vi "Analog Current Input - 1 Channel - Continuous Sampling.vi"() -> ()   [LabVIEW 2019]
uses:
  <vilib>/myRIO/Common/Instrument Driver Framework/myRIO v1.0/UART/vis/myRIO v1.0 Close UART.vi
  <vilib>/myRIO/Instrument Drivers/Onboard IO/AI Continuous/vis/AI Continuous Smart Read.vi
  <vilib>/myRIO/Common/Instrument Driver Framework/Utilities/vis/FPGA Ref Manager.vi
  <vilib>/myRIO/Common/Instrument Driver Framework/ELVIS III v1.0/ELVIS III v1.0 Reset FPGA.vi
  <vilib>/myRIO/Common/Instrument Driver Framework/myRIO v1.0/IRQ/vis/myRIO v1.0 IRQ Info FGV.vi
  <vilib>/myRIO/Common/Instrument Driver Framework/myRIO v1.0/IRQ/vis/myRIO v1.0 Timer IRQ Info FGV.vi
  <vilib>/myRIO/Common/Instrument Driver Framework/myRIO v1.0/IRQ/vis/myRIO v1.0 ISR Agent.vi
  <vilib>/myRIO/Instrument Drivers/Utilities/vis/Reset Index.vi
  <vilib>/myRIO/Common/Instrument Driver Framework/myRIO v1.0/Resource Manager/vis/myRIO v1.0 Block Write Resource Manager.vi
  <vilib>/myRIO/Express VI/Onboard IO/AI/AI Express VI.xnode
  <vilib>/myRIO/Instrument Drivers/Utilities/Utilities.lvlib
  <vilib>/myRIO/Instrument Drivers/Onboard IO/AI Continuous/AI Continuous.lvlib
panel:
  in  "电阻数值":dbl=1000.0 format="%#_6p"
  out "Analog Data":dbl[](graph)
  in  "Stop":bool
  # "ELVIS III Control IO"
  # "模拟输入单通道连续采样"
  # "Overview: Acquires current values continuously from Bank A, Channel 0 (A/AI0) until the acquisition is stopped.\nInstructions:\n1. Connect A/AI0 to a valid signal.\n2. Run the VI."
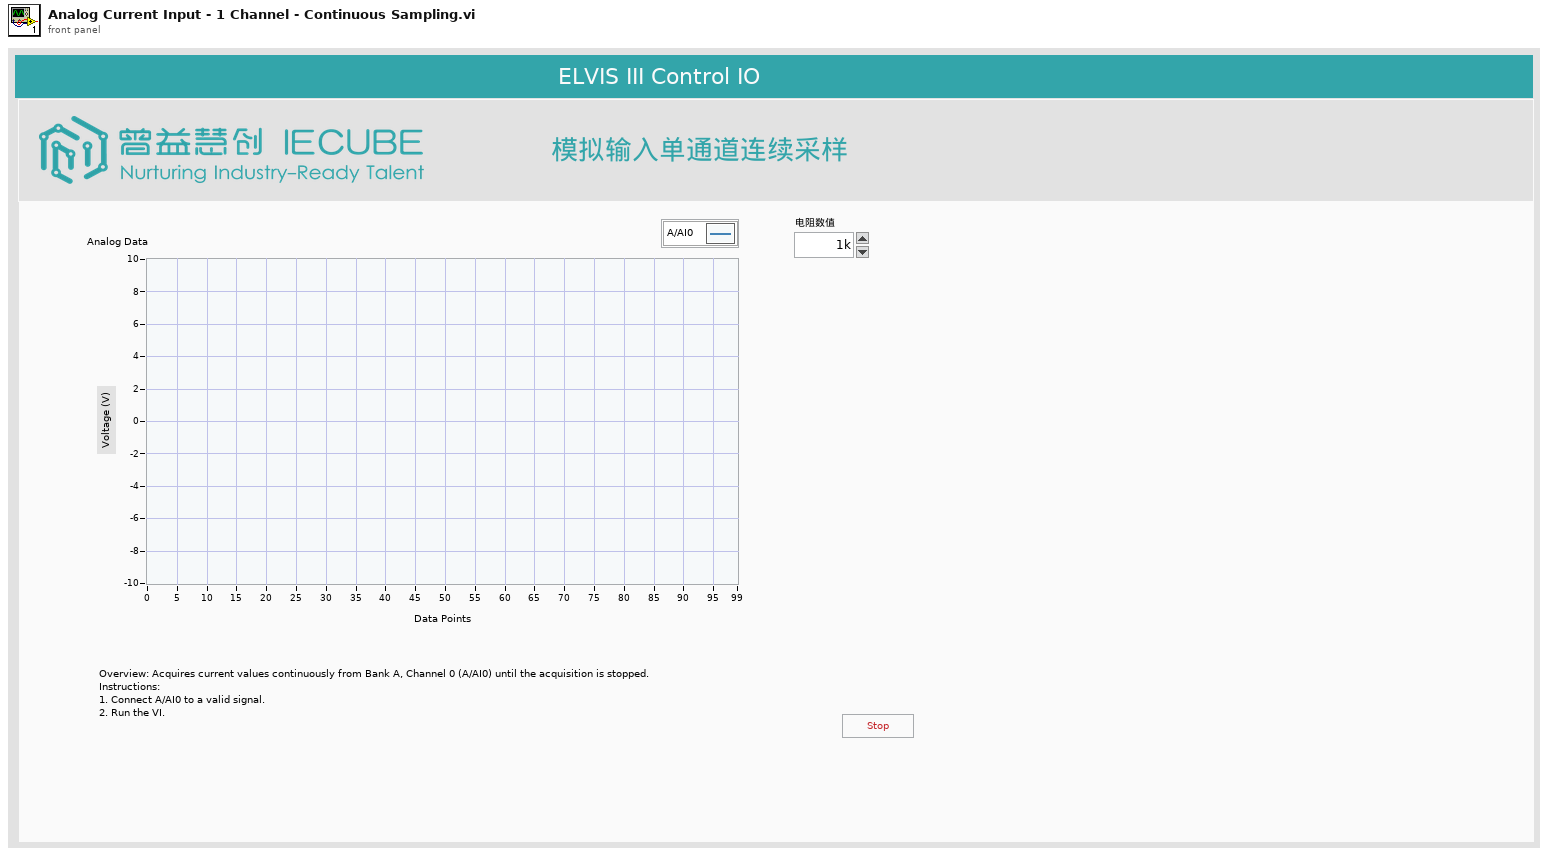
[diagram p1: front panel]
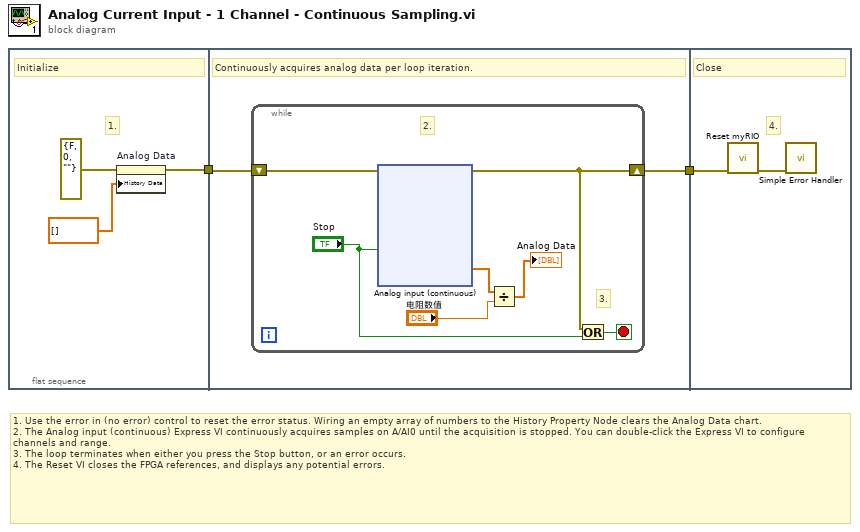
[diagram p0: block diagram]
diagram:
  # "1. Use the error in (no error) control to reset the error status. Wiring an empty array of numbers to the History Property Node clears the Analog Data chart.\n2. The Analog input (continuous) Express VI continuously acquires samples on A/AI0 until the acquisition is stopped. You can double-click the Express VI to configure channels and range.\n3. The loop terminates when either you press the Stop button, or an error occurs.\n4. The Reset VI closes the FPGA references, and displays any potential errors."
  n1 = flat-sequence {
    tunnel: [w3] -> w1
    tunnel: [w7] -> w2
    tunnel: w1 -> [w6]
    tunnel: w2 -> [w26]
    frame #0 {
      # "1."
      # "Initialize"
      n2 = property on="Analog Data" class="WFChart (严格)"(error in=errorcluster {"status"=FALSE, "code"=0, "source"=""} ("error constant"), "History Data"=dbl[] []) -> (error out=w3:errorcluster)  [unwired: 1 in, 1 out]
    }
    frame #1 {
      # "Continuously acquires analog data per loop iteration."
      n3 = while {
        shift-right: [w11] -> w7
        shift-left: w6 -> [w13]
        stop <- w12 stop-if-true
        # "3."
        # "2."
        n4 = xnode "Analog input (continuous)"("Stop?"="Stop", "error in (no error)"=w13) -> ("A/AI0 (Continuous)"=w10:dbl[], "error out"=w11:errorcluster)
        n5 = Divide(x=w10, y="电阻数值") -> (x/y=→"Analog Data":dbl[])
        n6 = Or(x=w11, y="Stop") -> (x .or. y?=w12:bool)
      }
    }
    frame #2 {
      # "4."
      # "Close"
      n7 = call <vilib>:"Reset myRIO.vi"("error in (no error)"=w26) -> ("error out"=w27:errorcluster)  [unwired: 10 in]
      n8 = call <vilib>:"Simple Error Handler.vi"("error in (no error)"=w27) -> ()  [unwired: 4 in, 5 out]
    }
  }
